vi "solar_voy_def Export (Item).vi"(10 "CMD":enum8{"CMD", "TLM"}(ring), 11 "ITEM":T2) -> (1 "Last Value (ASCII)":string, 2 "TYPE":T1, 3 "ITEM_DEF":string)   [LabVIEW 2018]
doc: "This exports a COSMOS definition parameter/item to string."
uses:
  solar_voy_def_ctl MODIFIERS LIMITS.ctl
  solar_voy_def_ctl MODIFIERS UNITS.ctl
  solar_voy_def_ctl MODIFIERS STATE.ctl
  solar_voy_def_ctl MODIFIERS CONVERSION.ctl
  solar_voy_def_ctl MODIFIERS.ctl
  solar_voy_def_ctl ITEM.ctl
  solar_voy_def_ctl ITEM TYPE.ctl
  type/solar_type Item Type.ctl
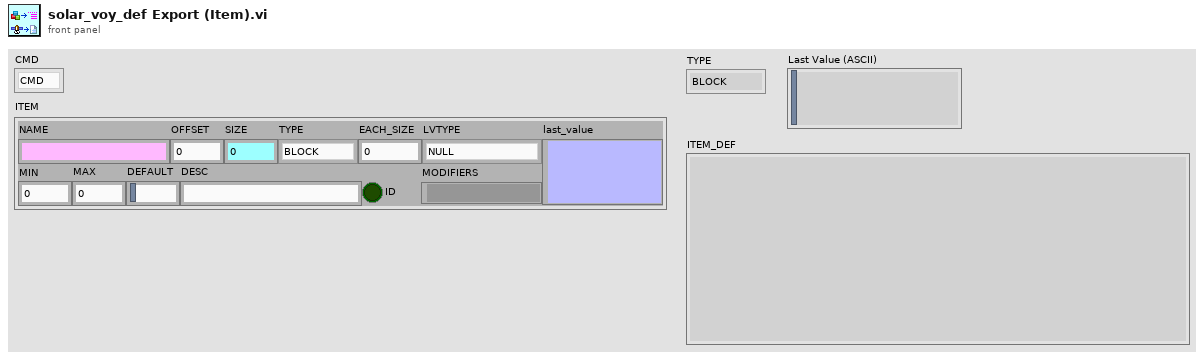
[diagram p1: front panel]
types:
  T1 = typedef "solar_voy_def_ctl ITEM TYPE.ctl" = enum8{"BLOCK", "INT", "UINT", "FLOAT", "STRING"}
  T2 = typedef "solar_voy_def_ctl ITEM.ctl" = cluster{"NAME":string, "OFFSET":i32, "SIZE":i32, "TYPE":T1, "EACH_SIZE":i32, "LVTYPE":T3, "MIN":dbl, "MAX":dbl, "DEFAULT":string, "DESC":string, "ID":bool, "MODIFIERS":variant, "last_value":variant}
  T3 = typedef "solar_type Item Type.ctl" = enum16{"NULL", "UNKNOWN", "CLUSTER", "I8", "I16", "I32", "I64", "U8", "U16", "U32", "U64", "U8_ENUM", "U16_ENUM", "U32_ENUM", "SGL", "DBL", "BOOLEAN", "STRING", "PATH", "VISA", "TAG", "TIME", "I8_1D", "I16_1D", "I32_1D", "I64_1D", "U8_1D", "U16_1D", "U32_1D", "U64_1D", "U8_ENUM_1D", "U16_ENUM_1D", "U32_ENUM_1D", "SGL_1D", "DBL_1D", "BOOLEAN_1D", "STRING_1D", "PATH_1D", "VISA_1D", "TAG_1D", "TIME_1D", "I8_2D", "I16_2D", "I32_2D", "I64_2D", "U8_2D", "U16_2D", "U32_2D", "U64_2D", "U8_ENUM_2D", "U16_ENUM_2D", "U32_ENUM_2D", "SGL_2D", "DBL_2D", "BOOLEAN_2D", "STRING_2D", "PATH_2D", "VISA_2D", "TAG_2D", "TIME_2D"}
  T4 = typedef "solar_voy_def_ctl MODIFIERS.ctl" = cluster{"LIMITS":T5, "UNITS":T6, "STATES":T7[], "CONVERSION":T8, "FORMAT":string, "REQUIRED":bool, "META":string[][]}
  T5 = typedef "solar_voy_def_ctl MODIFIERS LIMITS.ctl" = cluster{"NAME":string, "PERSIST":i32, "EN":bool, "RED_LO":dbl, "YEL_LO":dbl, "YEL_HI":dbl, "RED_HI":dbl, "GRN_LO":dbl, "GRN_HI":dbl, "FILENAME":string, "ARGS":string}
  T6 = typedef "solar_voy_def_ctl MODIFIERS UNITS.ctl" = cluster{"FULL":string, "ABV":string}
  T7 = typedef "solar_voy_def_ctl MODIFIERS STATE.ctl" = cluster{"KEY":string, "VALUE":string, "COLOR":string, "DESC":string, "HZRD":bool}
  T8 = typedef "solar_voy_def_ctl MODIFIERS CONVERSION.ctl" = cluster{"GENERIC":string, "FILENAME":string, "ARGS":string, "POLYS":cluster{"SEG":bool, "POLY":dbl[]}[]}
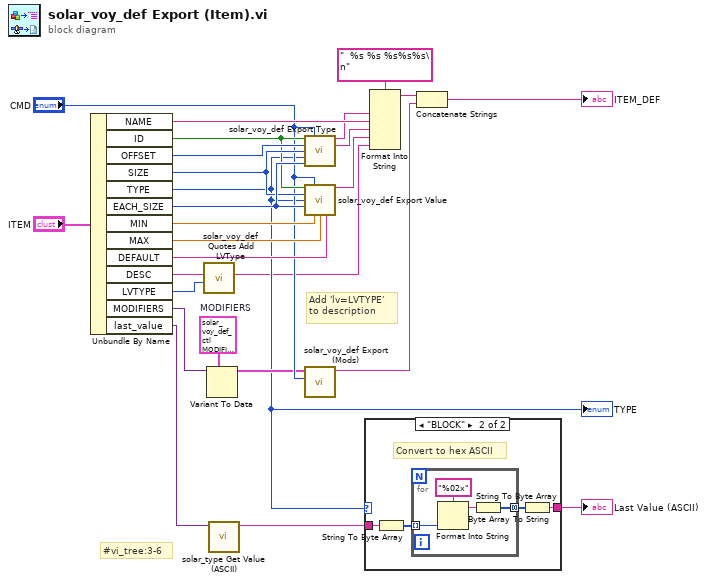
[diagram p0: block diagram]
diagram:
  w10 = T4 {"LIMITS"={"NAME"="", "PERSIST"=0, "EN"=FALSE, "RED_LO"=0.0, "YEL_LO"=0.0, "YEL_HI"=0.0, "RED_HI"=0.0, "GRN_LO"=0.0, "GRN_HI"=0.0, "FILENAME"="", "ARGS"=""}, "UNITS"={"FULL"="", "ABV"=""}, "STATES"=[], "CONVERSION"={"GENERIC"="", "FILENAME"="", "ARGS"="", "POLYS"=[]}, "FORMAT"="", "REQUIRED"=FALSE, "META"=[]}  # MODIFIERS
  # "#vi_tree:3-6"
  # "Add 'lv=LVTYPE'\nto description"
  n1 = Unbundle By Name("ITEM") -> ("NAME"=w23:string, "ID"=w12:bool, "OFFSET"=w21:i32, "SIZE"=w13:i32, "TYPE"=w4:T1, "EACH_SIZE"=w14:i32, "MIN"=w15:dbl, "MAX"=w16:dbl, "DEFAULT"=w17:string, "DESC"=w3:string, "LVTYPE"=w1:T3, "MODIFIERS"=w9:variant, "last_value"=w7:variant)
  "TYPE" <- w4
  n2 = call "solar_voy_def Quotes Add LVType.vi"("LVTYPE"=w1, "DESC in"=w3) -> ("DESC out"=w2:string)  [unwired: 9 in]
  n3 = Variant To Data(type=w10, Variant=w9) -> (data=w8:T4)  [unwired: 1 in, 1 out]
  n4 = call "solar_type Get Value (ASCII).vi"("Variant"=w7) -> ("Value (ASCII)"=w6:string)  [unwired: 8 in, 2 out]
  n5 = call "solar_voy_def Export Type.vi"("ID (F)"=w12, "CMD"="CMD", "OFFSET (-1=APPEND)"=w21, "TOTAL_SIZE (0)"=w13, "TYPE (BLOCK)"=w4, "EACH_SIZE (0=NoArray)"=w14) -> ("COMMAND_DEF"=w20:string, "TYPE_DEF"=w19:string)  [unwired: 8 in]
  n6 = call "solar_voy_def Export Value.vi"("ID"=w12, "CMD"="CMD", "SIZE"=w13, "TYPE"=w4, "EACH_SIZE (0=NoArray)"=w14, "MIN (NaN=Min)"=w15, "MAX (NaN=Max)"=w16, "DEFAULT (\"\"=Default)"=w17) -> ("VALUE_DEF"=w18:string)  [unwired: 7 in]
  n7 = call "solar_voy_def Export (Mods).vi"("CMD"="CMD", "MODIFIERS"=w8) -> ("MODIFIERS_DEF"=w24:string)  [unwired: 9 in]
  n8 = case shown="\"BLOCK\"" w4 {
    tunnel: w6 -> [w28 w30]
    tunnel: [w28 w29] -> w5
    frame Default {
    }
    frame "BLOCK" {
      # "Convert to hex ASCII"
      n9 = String To Byte Array(string=w30) -> (unsigned byte array=w32:u8[])
      n10 = for {
        tunnel: w32 -> [w36] mode=indexing
        tunnel: [w33] -> w31 mode=concatenating
        n11 = Format Into String(format string="%02x" ("Format String"), w36) -> (resulting string=w34:string)  [unwired: 2 in, 1 out]
        n12 = String To Byte Array(string=w34) -> (unsigned byte array=w33:u8[])
      }
      n13 = Byte Array To String(unsigned byte array=w31) -> (string=w29:string)
    }
  }
  "Last Value (ASCII)" <- w5
  n14 = Format Into String(format string="  %s %s %s%s%s\n", w20, w23, w19, w18, w2) -> (resulting string=w26:string)  [unwired: 2 in, 1 out]
  n15 = Concatenate Strings(w26, w24) -> (→"ITEM_DEF":string)
